vi "Add_Part_of_Track(After_101)_Problem-1.vi"(4 "[IN] Index in subtrack":i32, 5 "[IN] Minimal Sub\ntrack Length":i32, 6 "[IN] Subtrack":T2, 7 "[IN] Indexes for Jumps":i32[](array[numeric]), 8 "error IN":errorcluster, 9 "[IN] Count of variants":i32, 10 "[IN] Subtracks":T1(array[cluster]), 11 "[IN] Still connected\ntracks in group":T3) -> (0 "error OUT":errorcluster, 1 "[OUT] Count of variants":i32, 2 "[OUT] Subtracks":T1(array[cluster]))   [LabVIEW 2013]
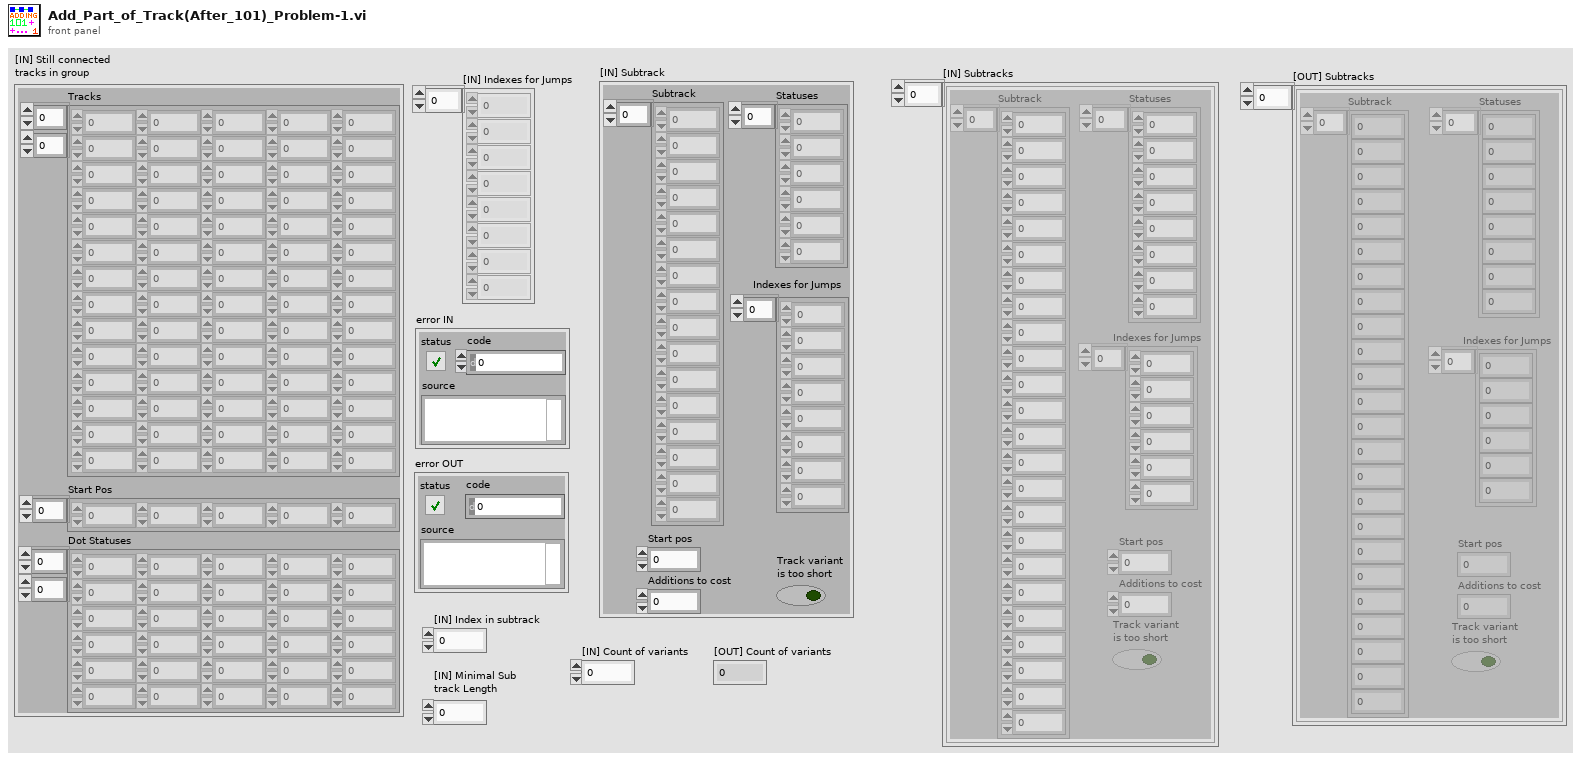
[diagram p1: front panel]
types:
  T1 = cluster{"Subtrack":dbl[], "Statuses":i16[], "Start pos":i32, "Additions to cost":i32, "Track variant \nis too short":bool, "Indexes for Jumps":i32[]}[]
  T2 = cluster{"Subtrack":dbl[], "Statuses":i16[], "Start pos":i32, "Additions to cost":i32, "Track variant \nis too short":bool, "Indexes for Jumps":i32[]}
  T3 = cluster{"Tracks":dbl[][], "Start Pos":i32[], "Dot Statuses":i16[][]}
  T4 = cluster{"Subtrack":dbl[], "Statuses":i16[], "Start pos":i32, "Additions to cost":i8, "Track variant \nis too short":bool, "Indexes for Jumps":i32[]}
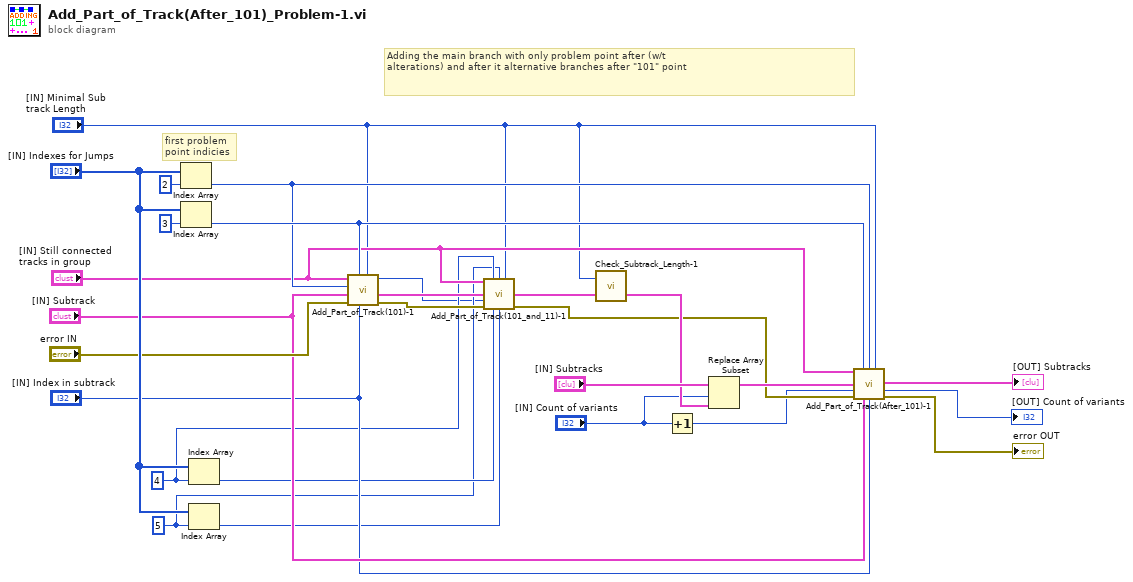
[diagram p0: block diagram]
diagram:
  w2 = 5 ("index")
  w4 = 4 ("index")
  # "first problem \npoint indicies"
  # "Adding the main branch with only problem point after (w/t \nalterations) and after it alternative branches after \"101\" point"
  n1 = Index Array(array="[IN] Indexes for Jumps", index=2) -> (element=w14:i32)
  n2 = Index Array(array="[IN] Indexes for Jumps", index=3) -> (element=w15:i32)
  n3 = Index Array(array="[IN] Indexes for Jumps", index=w4) -> (element=w6:i32)
  n4 = Index Array(array="[IN] Indexes for Jumps", index=w2) -> (element=w5:i32)
  n5 = call "Add_Part_of_Track(101)-1.vi"("[IN] Minimal Sub\ntrack Length"="[IN] Minimal Sub\ntrack Length", "[IN] Index in subtrack"="[IN] Index in subtrack", "[IN] # of subtrack conta\nining problem point"=w15, "error IN"="error IN", "[IN] Subtrack"="[IN] Subtrack", "[IN] Index of problem\npoint inside subtrack"=w14, "[IN] Still connected\ntracks in group"="[IN] Still connected\ntracks in group") -> ("error OUT"=w9:errorcluster, "[OUT] Subtrack"=w10:T2, "[OUT] Last point in subtrack"=w1:i32)  [unwired: 2 in]
  n6 = call "Add_Part_of_Track(101_and_11)-1.vi"("[IN] Still connected\ntracks in group"="[IN] Still connected\ntracks in group", "[IN] i for Probl\nem  Point Index"=w4, "[IN] i for # of Track \nwith Problem Point"=w2, "[IN] Minimal Sub\ntrack Length"="[IN] Minimal Sub\ntrack Length", "[IN] Subtrack"=w10, "[IN] Index in subtrack"=w1, "error IN"=w9, "[IN] Index of problem\npoint inside subtrack"=w6, "[IN] # of subtrack conta\nining problem point"=w5) -> ("[OUT] Subtrack"=w23:T2, "error OUT"=w18:errorcluster)  [unwired: 4 in, 1 out]
  n7 = call "Check_Subtrack_Length-1.vi"("[IN] Subtrack"=w23, "[IN] Minimal Sub\ntrack Length"="[IN] Minimal Sub\ntrack Length") -> ("[OUT] Subtrack"=w21:T4)  [unwired: 1 in]
  n8 = Increment(x="[IN] Count of variants") -> (x+1=w17:i32)
  n9 = Replace Array Subset(array="[IN] Subtracks", new element=w21, index="[IN] Count of variants") -> (w19:T1)
  n10 = call "Add_Part_of_Track(After_101)-1.vi"("[IN] Still connected\ntracks in group"="[IN] Still connected\ntracks in group", "[IN] # of subtrack conta\nining problem point"=w15, "[IN] Index of problem\npoint inside subtrack"=w14, "[IN] Minimal Sub\ntrack Length"="[IN] Minimal Sub\ntrack Length", "[IN] Subtracks"=w19, "[IN] Count of variants"=w17, "error IN"=w18, "[IN] Subtrack"="[IN] Subtrack", "[IN] Index in subtrack"="[IN] Index in subtrack") -> ("[OUT] Subtracks"=→"[OUT] Subtracks":T1, "[OUT] Count of variants"=→"[OUT] Count of variants":i32, "error OUT"=→"error OUT":errorcluster)  [unwired: 4 in]
